vi "MyrioProject.vi"() -> ()   [LabVIEW 2018]
doc: "The myRIO Project template acquires acceleration data from the onboard accelerometer and displays the changes of acceleration values in a waveform chart."
uses:
  <vilib>/myRIO/Common/Instrument Driver Framework/Utilities/typedefs/Generic FPGA Reference.ctl
  <vilib>/myRIO/Common/Instrument Driver Framework/Utilities/typedefs/myRIO v1.0 Reference.ctl
  <vilib>/myRIO/Common/Instrument Driver Framework/Utilities/typedefs/Hardware Version Enum.ctl
  <vilib>/myRIO/Common/Instrument Driver Framework/Utilities/typedefs/myRIO Generic Hardware Reference.ctl
  <vilib>/userdefined/High Color/nirio_resource_hc.ctl
  <vilib>/myRIO/Common/Instrument Driver Framework/myRIO v1.0/Encoder/typedefs/Encoder Channels Enum.ctl
  <vilib>/myRIO/Instrument Drivers/Onboard IO/Encoder/typedefs/Encoder Reference.ctl
  <vilib>/myRIO/Instrument Drivers/Onboard IO/Encoder/Encoder.lvlib
  <vilib>/myRIO/Common/Instrument Driver Framework/myRIO v1.0/Encoder/typedefs/Encoder Signal Mode.ctl
  <vilib>/myRIO/Instrument Drivers/Onboard IO/Encoder/vis/myRIO Encoder Open.xnode
  <vilib>/myRIO/Common/Instrument Driver Framework/myRIO v1.0/Encoder/vis/myRIO v1.1 Open Encoder.vi
  <vilib>/myRIO/Common/Instrument Driver Framework/myRIO v1.0/Encoder/vis/myRIO v1.0 Configure Encoder.vi
  <vilib>/myRIO/Common/Instrument Driver Framework/myRIO v1.0/Encoder/typedefs/Encoder Configuration v1.0.ctl
  <vilib>/myRIO/Instrument Drivers/Onboard IO/PWM/typedefs/PWM Configuration.ctl
  <vilib>/myRIO/Instrument Drivers/Onboard IO/PWM/PWM.lvlib
  <vilib>/myRIO/Common/Instrument Driver Framework/myRIO v1.0/PWM/typedefs/PWM Channels Enum.ctl
  <vilib>/myRIO/Instrument Drivers/Onboard IO/PWM/typedefs/PWM Reference.ctl
  <vilib>/myRIO/Instrument Drivers/Onboard IO/PWM/vis/myRIO PWM Open.xnode
  <vilib>/myRIO/Common/Instrument Driver Framework/myRIO v1.0/PWM/vis/myRIO v1.1 Open PWM.vi
  <vilib>/myRIO/Express VI/Onboard Devices/Button/Button Express VI.xnode
  <vilib>/myRIO/Instrument Drivers/Onboard IO/DIO/typedefs/DIO Reference.ctl
  <vilib>/myRIO/Instrument Drivers/Onboard IO/DIO/DIO.lvlib
  <vilib>/myRIO/Common/Instrument Driver Framework/myRIO v1.0/DIO/typedefs/DIO Channels List.ctl
  <vilib>/myRIO/Common/Instrument Driver Framework/myRIO v1.0/DIO/typedefs/DIO Channels Enum.ctl
  <vilib>/myRIO/Instrument Drivers/Onboard IO/DIO/vis/myRIO DIO Open.xnode
  <vilib>/myRIO/Common/Instrument Driver Framework/myRIO v1.0/DIO/vis/myRIO v1.1 Open DIO.vi
  <vilib>/myRIO/Common/Instrument Driver Framework/Utilities/vis/Is FPGA Ref Available.vi
  <vilib>/myRIO/Express VI/Onboard IO/DO/DO Express VI.xnode
  <vilib>/myRIO/Instrument Drivers/Onboard IO/DIO/vis/Write.vi
  <vilib>/myRIO/Express VI/Onboard IO/AI/AI Express VI.xnode
  <vilib>/myRIO/Instrument Drivers/Onboard IO/AI/typedefs/AI Reference.ctl
  <vilib>/myRIO/Instrument Drivers/Onboard IO/AI/AI.lvlib
  <vilib>/myRIO/Common/Instrument Driver Framework/Utilities/typedefs/Analog Scaling Constants List.ctl
  <vilib>/myRIO/Common/Instrument Driver Framework/Utilities/typedefs/Analog Scaling Constants.ctl
  <vilib>/myRIO/Common/Instrument Driver Framework/myRIO v1.0/AI/typedefs/AI Channels List.ctl
  <vilib>/myRIO/Common/Instrument Driver Framework/myRIO v1.0/AI/typedefs/AI Channels Enum.ctl
  <vilib>/myRIO/Instrument Drivers/Onboard IO/AI/vis/myRIO AI Open.xnode
  <vilib>/myRIO/Common/Instrument Driver Framework/myRIO v1.0/AI/vis/myRIO v1.1 Open AI.vi
  <vilib>/myRIO/Express VI/Onboard IO/PWM/PWM Express VI.xnode
  <vilib>/myRIO/Instrument Drivers/Onboard IO/PWM/vis/Set Duty Cycle and Frequency.vi
  <vilib>/platform/TimedLoop/XDataNode/XDataNode.xnode
  <vilib>/Platform/TimedLoop/XDataNode/timing_clust.ctl
  <vilib>/Platform/TimedLoop/XDataNode/XDNodeRunTimeDep.lvlib
  <vilib>/Platform/TimedLoop/XDataNode/wakeup.ctl
  <vilib>/Platform/TimedLoop/XDataNode/nitl_modes.ctl
panel:
  out "Numeric Control":dbl
  out "data":dbl
  out "Double 2":dbl
  out "Double":dbl
  out "sensor2 (A/AI2 (Pin 7))":dbl
  out "sensor1":dbl
  out "stallRojo (A/AI0 (Pin 3))":dbl
  out "stallBlanco (A/AI1 (Pin 5))":dbl
  in  "MANUAL 2":bool
  in  "Stop Button":bool
  in  "Start":bool
  out "element":dbl
  out "element 2":dbl
  out "subarray 2":dbl[][](array[numeric])
  out "subarray":dbl[][](array[numeric])
  out "vectores":dbl[][][](array[numeric])
  in  "saturacion":dbl=0.3
  in  "Duty Cycle 2":dbl(slide)=0.5 scale=0.05..0.1
  in  "Duty Cycle":dbl(slide)=0.5 scale=0.05..0.1
  in  "Reset Counter 2":bool
  in  "Reset Counter":bool
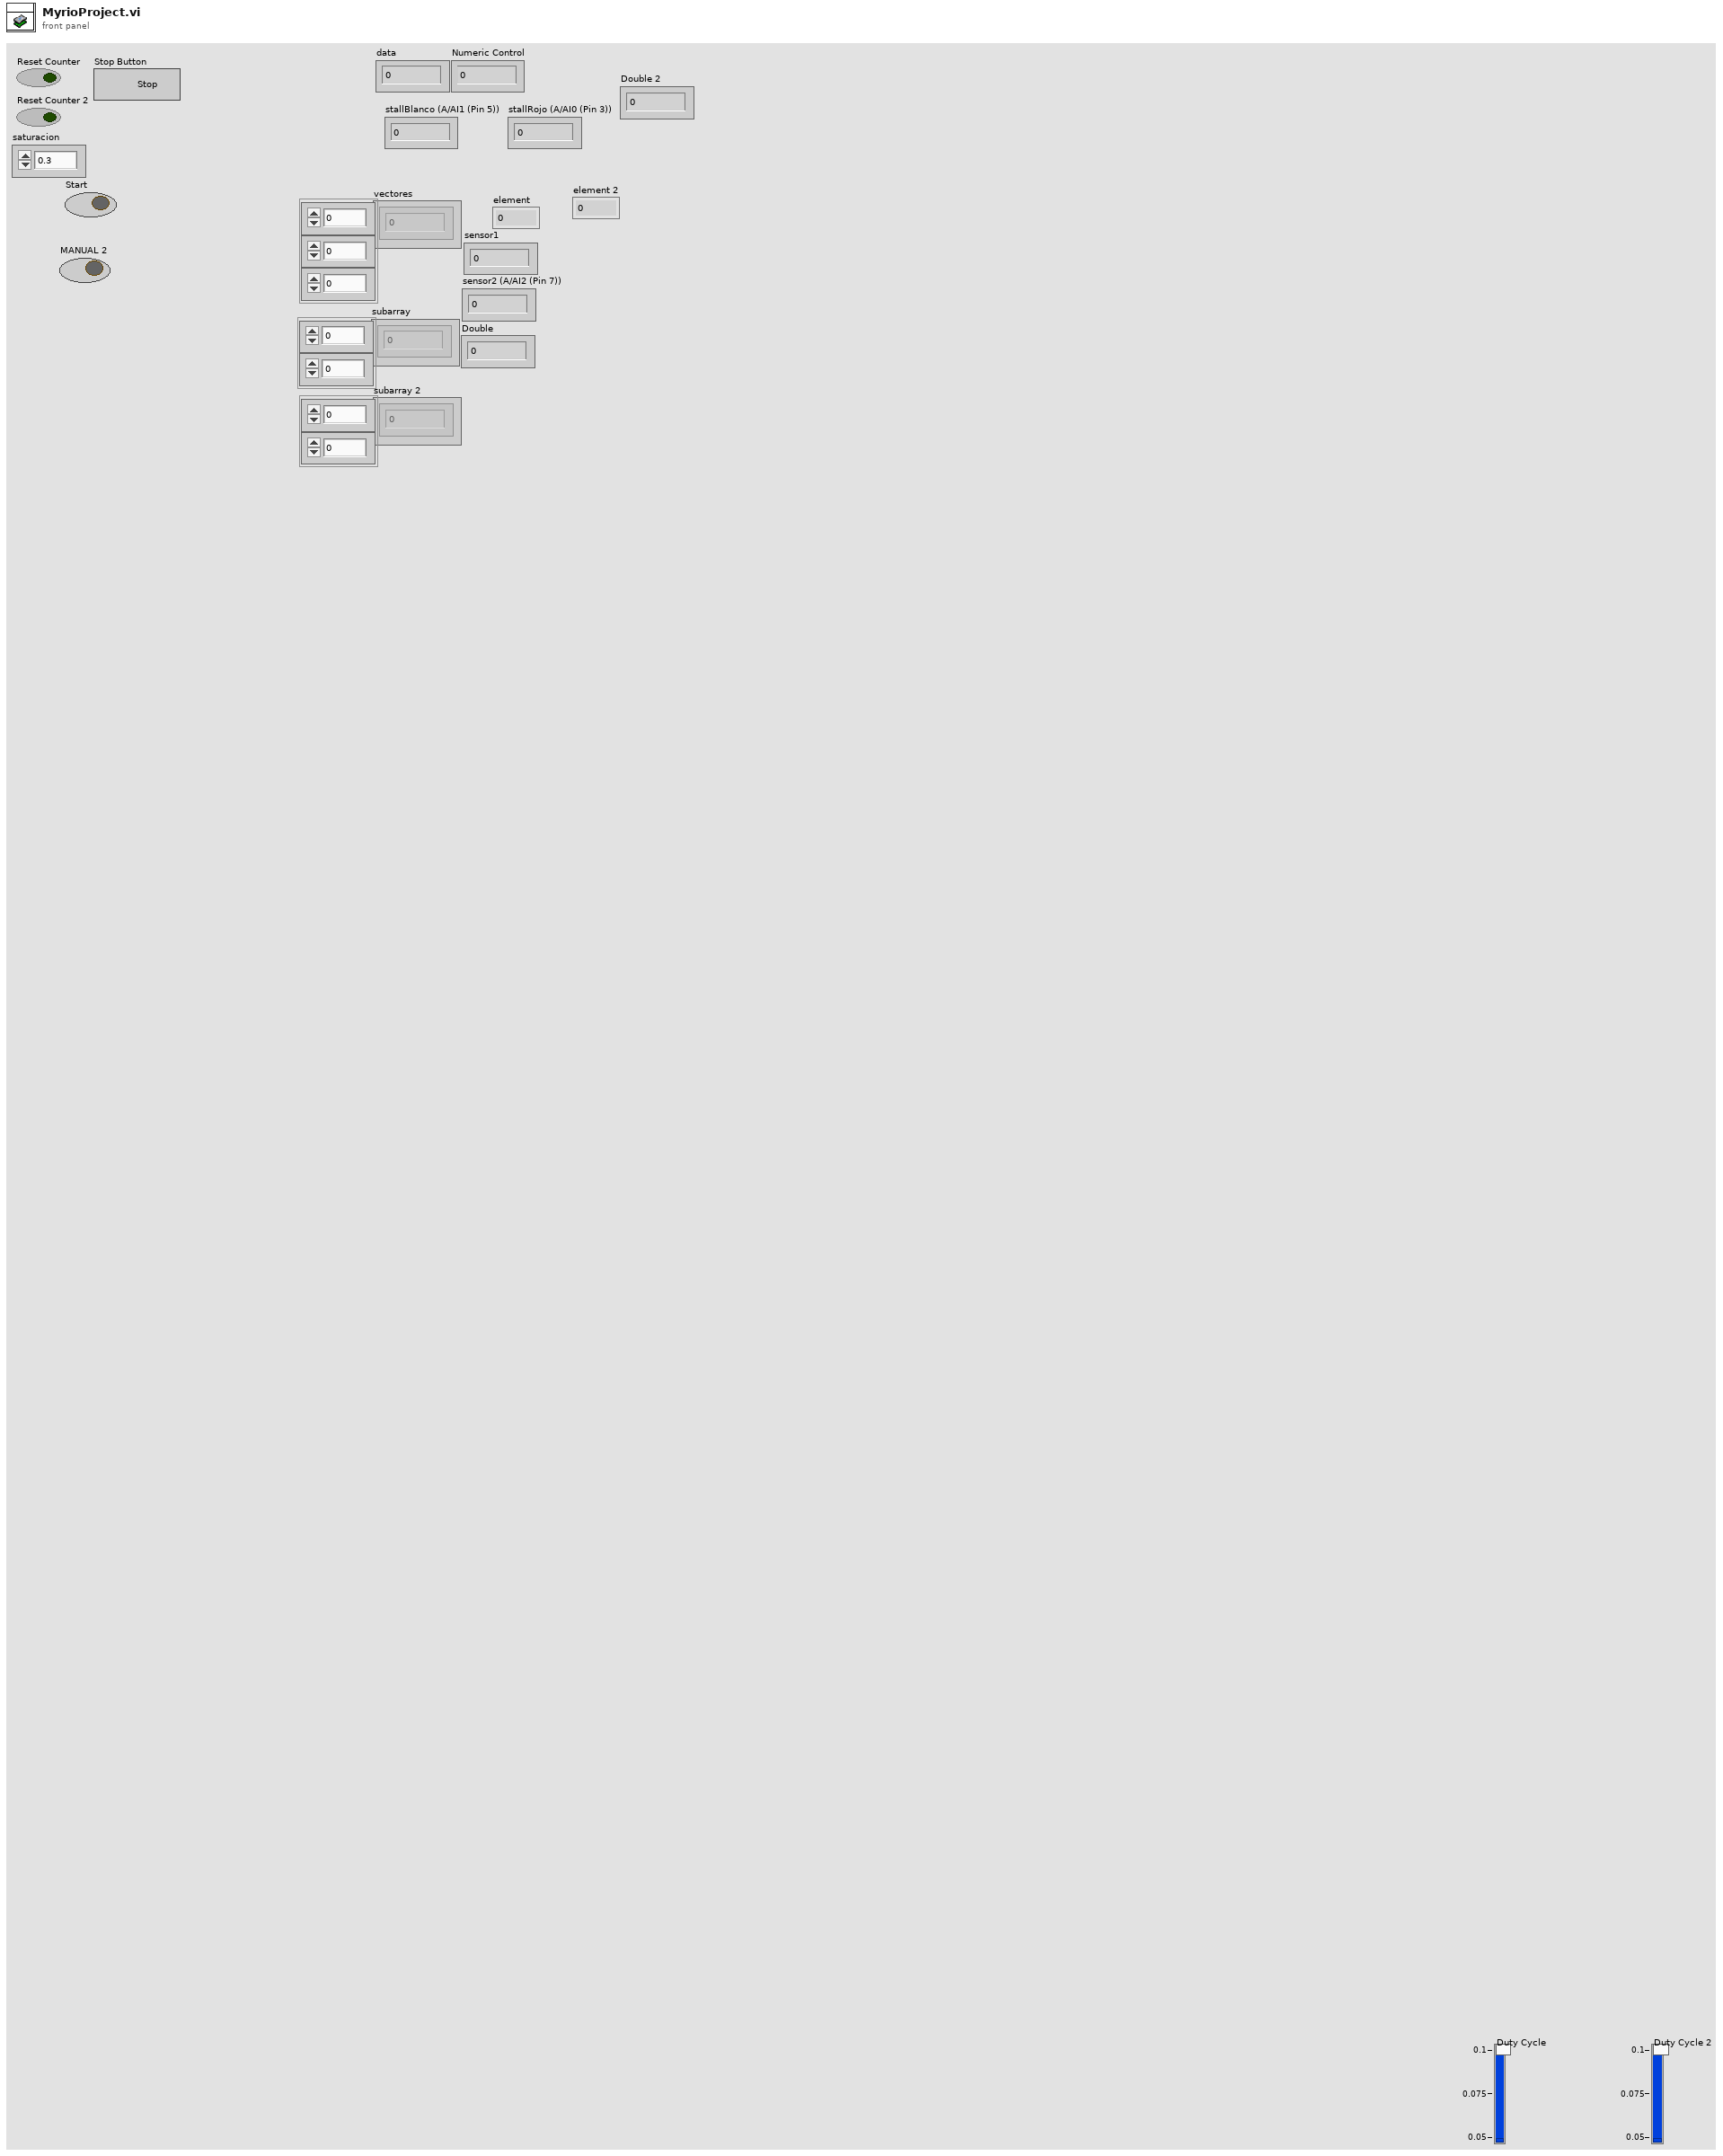
[diagram p1: front panel]
types:
  T1 = enum16{"normal", "grande-Sensor", "grande home", "peque-sensor", "peque- home", "peque-reset"}
  T2 = typedef "Encoder Signal Mode.ctl" = enum16{"Quadrature phase signal", "Step and direction signal"}
  T3 = typedef "PWM.lvlib/PWM Reference.ctl" = cluster{"myRIO Reference":T4, "PWM Channels Enum":T8, "PWM Configuration":T9}
  T4 = typedef "myRIO Generic Hardware Reference.ctl" = cluster{"myRIO Model":T5, "myRIO Hardware Reference":T6}
  T5 = typedef "Hardware Version Enum.ctl" = enum16{"Unknown", "myRIO-1900", "myRIO-1950", "roboRIO", "NI ELVIS RIO CM", "ELVIS III"}
  T6 = typedef "myRIO v1.0 Reference.ctl" = cluster{"Generic FPGA Reference":T7, "Allow multiple opens":bool}
  T7 = typedef "Generic FPGA Reference.ctl" = refnum<k20>
  T8 = typedef "PWM Channels Enum.ctl" = enum16{"Not Connected", "C/PWM0", "C/PWM1", "A/PWM0", "A/PWM1", "A/PWM2", "A/PWM3", "A/PWM4", "A/PWM5", "A/PWM6", "A/PWM7", "A/PWM8", "A/PWM9", "A/PWM10", "A/PWM11", "A/PWM12", "A/PWM13", "A/PWM14", "A/PWM15", "A/PWM16", "A/PWM17", "A/PWM18", "A/PWM19", "B/PWM0", "B/PWM1", "B/PWM2", "B/PWM3", "B/PWM4", "B/PWM5", "B/PWM6", "B/PWM7", "B/PWM8", "B/PWM9", "B/PWM10", "B/PWM11", "B/PWM12", "B/PWM13", "B/PWM14", "B/PWM15", "B/PWM16", "B/PWM17", "B/PWM18", "B/PWM19", "PWM/PWM0", "PWM/PWM1", "PWM/PWM2", "PWM/PWM3", "PWM/PWM4", "PWM/PWM5", "PWM/PWM6", "PWM/PWM7", "PWM/PWM8", "PWM/PWM9"}
  T9 = typedef "PWM.lvlib/PWM Configuration.ctl" = cluster{"Frequency":dbl, "Duty Cycle":dbl}
  T10 = typedef "Encoder.lvlib/Encoder Reference.ctl" = cluster{"myRIO Reference":T4, "Encoder Channels Enum":T11}
  T11 = typedef "Encoder Channels Enum.ctl" = enum16{"Not Connected", "C/ENC0", "C/ENC1", "A/ENC", "A/ENC0", "A/ENC1", "A/ENC2", "A/ENC3", "A/ENC4", "A/ENC5", "A/ENC6", "A/ENC7", "A/ENC8", "A/ENC9", "B/ENC", "B/ENC0", "B/ENC1", "B/ENC2", "B/ENC3", "B/ENC4", "B/ENC5", "B/ENC6", "B/ENC7", "B/ENC8", "B/ENC9", "DIO/ENC0", "DIO/ENC1", "DIO/ENC2", "DIO/ENC3", "DIO/ENC4"}
  T12 = cluster{"Double":dbl, "dbl Scaled Value":dbl, "Output":dbl, "seconds since 1Jan1904":timestamp, dbl, dbl, dbl}
  T13 = typedef "XDNodeRunTimeDep.lvlib/timing_clust.ctl" = cluster{"Expected End [f-1]":u64, "Actual End [f-1]":u64, "Finished Late? [f-1]":bool, "Expected End [i-1]":u64, "Actual End [i-1]":u64, "Finished Late? [i-1]":bool, "Expected Start [i]":u64, "Actual Start [i]":u64, "Expected Start [f]":u64, "Actual Start [f]":u64, "Source Name":string, "Structure Name":string, "Period":i64, "Deadline":i64, "Offset":i64, "Start":i64, "Priority":i32, "Timeout":i32, "Mode":T14, "Wakeup Reason":T15, "Error":errorcluster, "Source Type":string, "Secondary Source Type":string, "Global End Time":u64, "Global Start Time":u64, "Frame Duration":u64, "Iteration Duration":u64, "Assigned CPU":i32, "I/O Scan Engine Mode":u32}
  T14 = typedef "XDNodeRunTimeDep.lvlib/nitl_modes.ctl" = enum32{"No Change", "Process missed periods, maintain original phase", "Discard missed periods, maintain original phase", "Process missed periods, ignore original phase", "Discard missed periods, ignore original phase"}
  T15 = typedef "XDNodeRunTimeDep.lvlib/wakeup.ctl" = enum32{"Normal", "Aborted", "Asynchronous wakeup", "Timing source error", "Timed loop error", "Timeout"}
  T16 = typedef "nirio_resource_hc.ctl" = tag
  T17 = typedef "AI.lvlib/AI Reference.ctl" = cluster{"myRIO Reference":T4, "AI Channels List":T18, "AI Scaling Constants List":T20}
  T18 = typedef "AI Channels List.ctl" = T19[]
  T19 = typedef "AI Channels Enum.ctl" = enum16{"Not Connected", "AudioIn/Left", "AudioIn/Right", "C/AI0", "C/AI1", "A/AI0", "A/AI1", "A/AI2", "A/AI3", "A/AI4", "A/AI5", "A/AI6", "A/AI7", "B/AI0", "B/AI1", "B/AI2", "B/AI3", "B/AI4", "B/AI5", "B/AI6", "B/AI7", "AI/AI0", "AI/AI1", "AI/AI2", "AI/AI3", "A/AI0 (DIFF)", "A/AI1 (DIFF)", "A/AI2 (DIFF)", "A/AI3 (DIFF)", "B/AI0 (DIFF)", "B/AI1 (DIFF)", "B/AI2 (DIFF)", "B/AI3 (DIFF)"}
  T20 = typedef "Analog Scaling Constants List.ctl" = T21[]
  T21 = typedef "Analog Scaling Constants.ctl" = cluster{"LSB Weight (Volts)":dbl, "Offset (Volts)":dbl, "Signed?":bool}
  T22 = typedef "DIO.lvlib/DIO Reference.ctl" = cluster{"myRIO Reference":T4, "DIO Channels List":T23}
  T23 = typedef "DIO Channels List.ctl" = T24[]
  T24 = typedef "DIO Channels Enum.ctl" = enum16{"Not Connected", "C/DIO0", "C/DIO1", "C/DIO2", "C/DIO3", "C/DIO4", "C/DIO5", "C/DIO6", "C/DIO7", "A/DIO0", "A/DIO1", "A/DIO2", "A/DIO3", "A/DIO4", "A/DIO5", "A/DIO6", "A/DIO7", "A/DIO8", "A/DIO9", "A/DIO10", "A/DIO11", "A/DIO12", "A/DIO13", "A/DIO14", "A/DIO15", "A/DIO16", "A/DIO17", "A/DIO18", "A/DIO19", "B/DIO0", "B/DIO1", "B/DIO2", "B/DIO3", "B/DIO4", "B/DIO5", "B/DIO6", "B/DIO7", "B/DIO8", "B/DIO9", "B/DIO10", "B/DIO11", "B/DIO12", "B/DIO13", "B/DIO14", "B/DIO15", "B/DIO16", "B/DIO17", "B/DIO18", "B/DIO19", "LED0", "LED1", "LED2", "LED3", "Button0", "DIO/DIO0", "DIO/DIO1", "DIO/DIO2", "DIO/DIO3", "DIO/DIO4", "DIO/DIO5", "DIO/DIO6", "DIO/DIO7", "DIO/DIO8", "DIO/DIO9", "SPI/CS0", "SPI/CS1", "SPI/CS2", "SPI/CS3", "LED RADIO (Green)", "LED RADIO (Red)", "LED COMM (Green)", "LED COMM (Red)", "LED MODE (Green)", "LED MODE (Red)"}
  T25 = cluster{dbl, void, "Counter Value":i32, "seconds since 1Jan1904":timestamp, dbl, "saturacion":dbl, "Counter Value":i32}
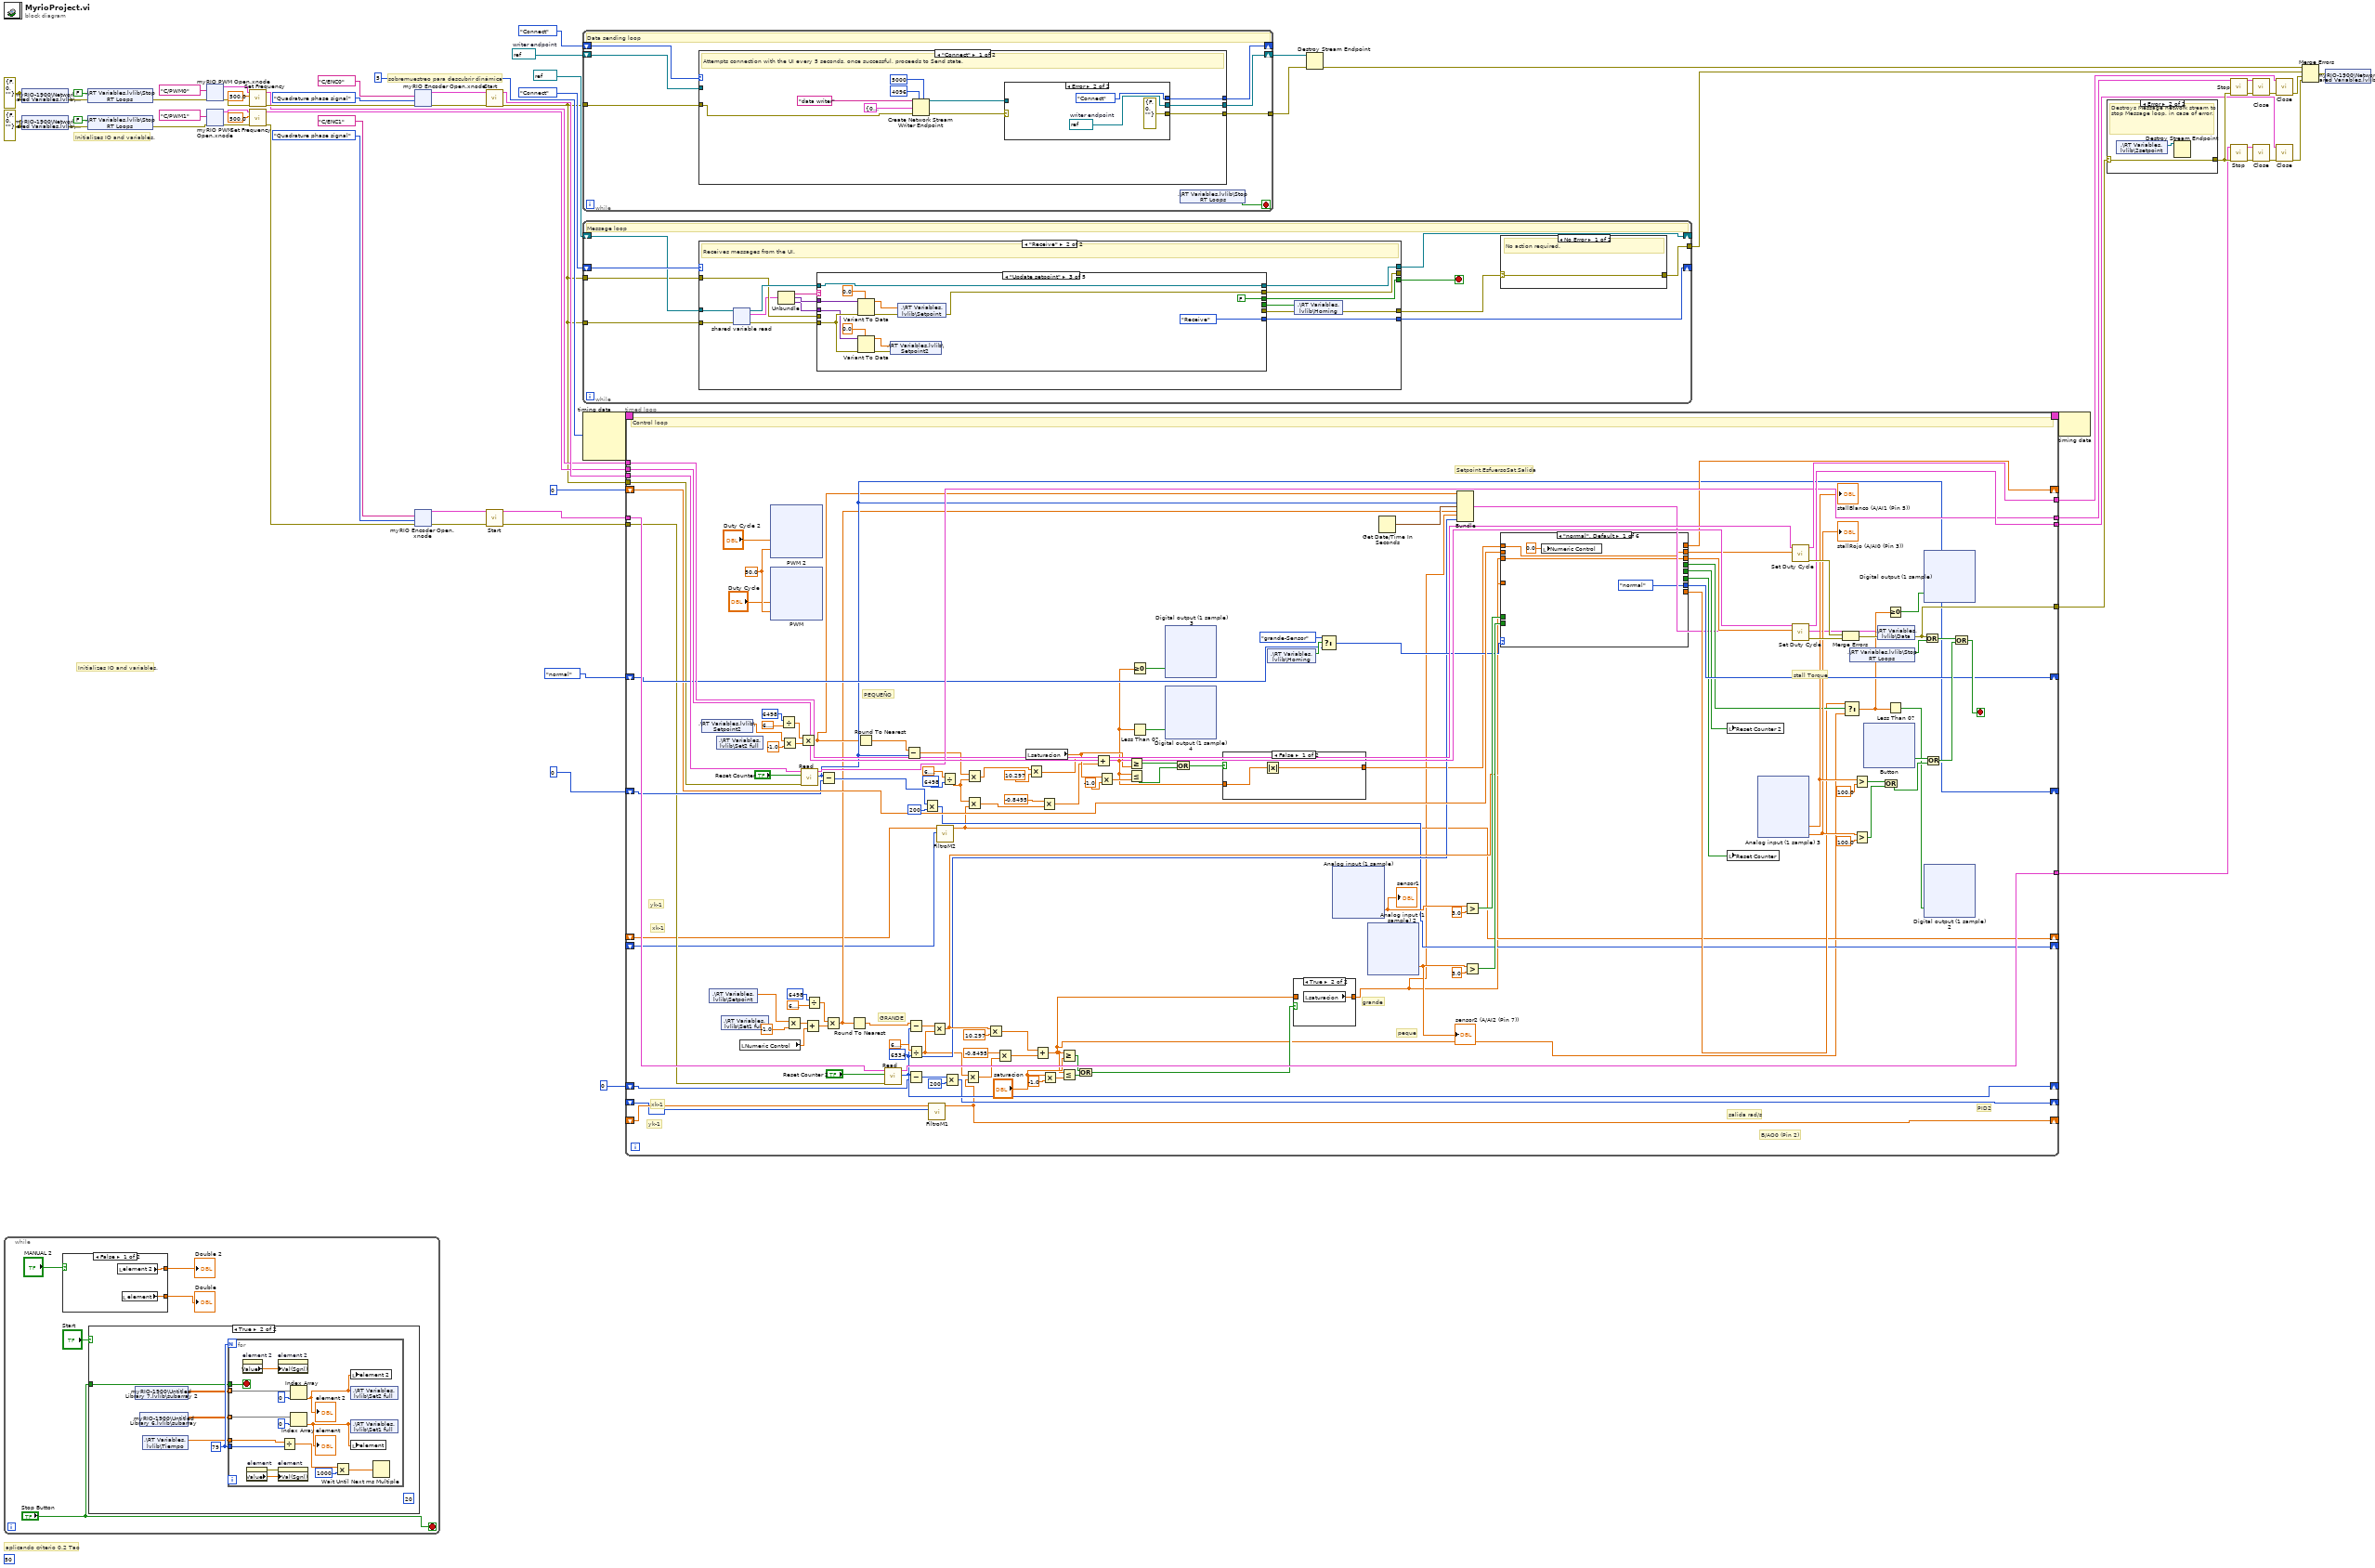
[diagram p0: block diagram]
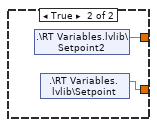
[diagram p2: hidden frame]
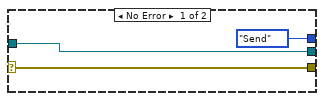
[diagram p5: hidden frame]
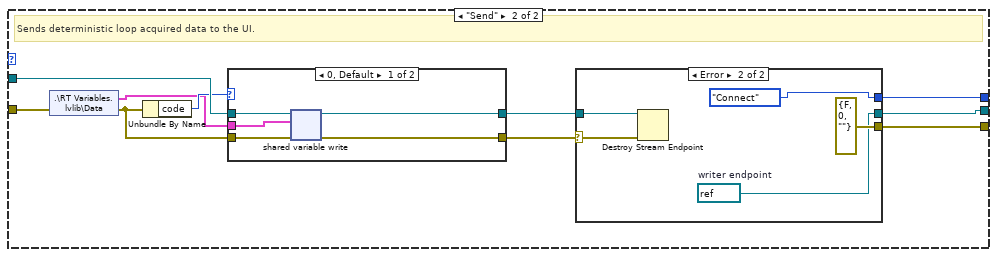
[diagram p6: hidden frame]
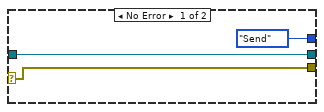
[diagram p7: hidden frame]
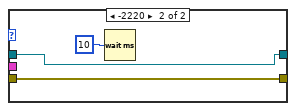
[diagram p8: hidden frame]
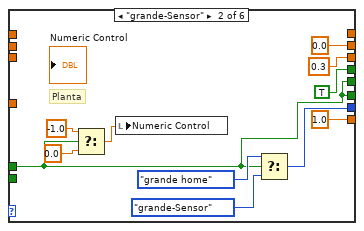
[diagram p9: hidden frame]
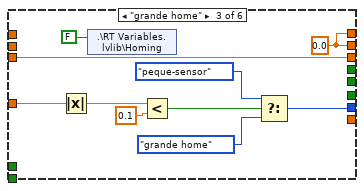
[diagram p10: hidden frame]
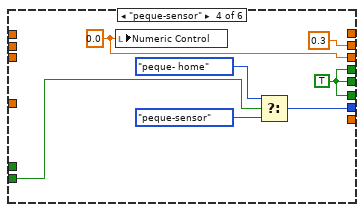
[diagram p11: hidden frame]
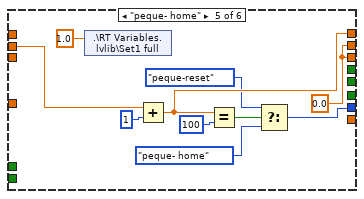
[diagram p12: hidden frame]
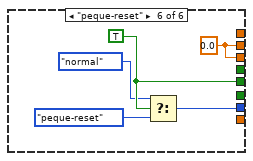
[diagram p13: hidden frame]
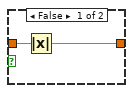
[diagram p14: hidden frame]
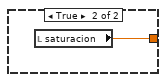
[diagram p15: hidden frame]
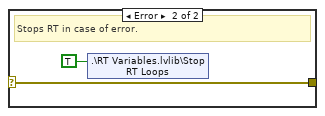
[diagram p16: hidden frame]
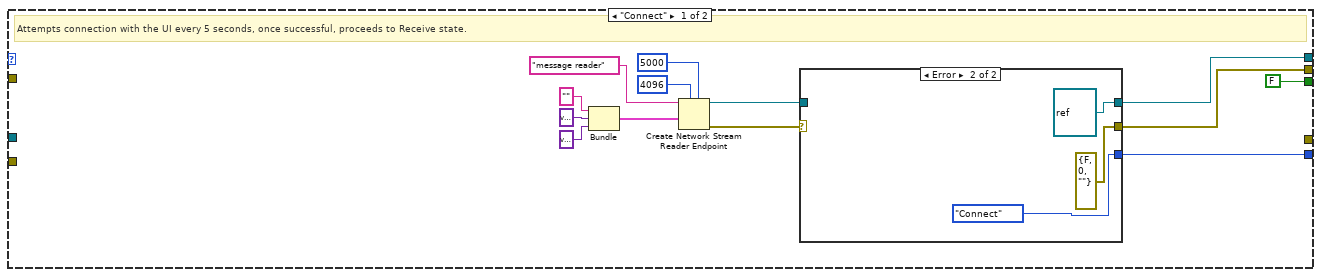
[diagram p17: hidden frame]
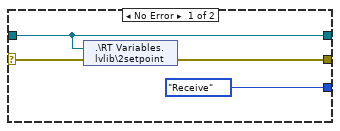
[diagram p18: hidden frame]
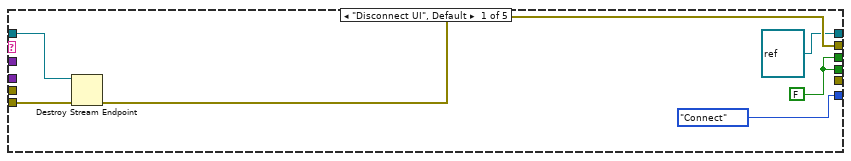
[diagram p19: hidden frame]
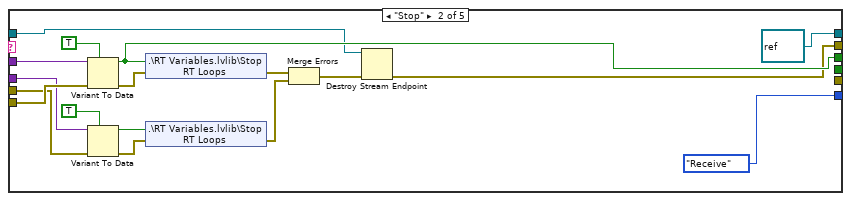
[diagram p20: hidden frame]
diagram:
  (unwired) 50
  w16 = refnum<k21> refnum  # writer endpoint
  w29 = errorcluster {"status"=FALSE, "code"=0, "source"=""} ("error IO")
  w51 = errorcluster {"status"=FALSE, "code"=0, "source"=""} ("error IO")
  # "aplicando criterio 0.2 Tao"
  # "sobremuestreo para descubrir dinámica"
  # "Initializes IO and variables."
  # "Initializes IO and variables."
  n1 = while {
    stop <- "Stop Button" stop-if-true
    n2 = case shown="False" "MANUAL 2" {
      tunnel: [w69 w71] -> w63
      tunnel: [w68 w70] -> w64
      frame False {
        n3 = local read "element 2"() -> (w69:dbl)
        n4 = local read "element"() -> (w68:dbl)
      }
      frame True {
        n5 = shared-variable ".\\RT Variables.lvlib\\Setpoint2"() -> (w71:dbl)  [unwired: 1 in, 1 out]
        n6 = shared-variable ".\\RT Variables.lvlib\\Setpoint"() -> (w70:dbl)  [unwired: 1 in, 1 out]
      }
    }
    "Double" <- w64
    "Double 2" <- w63
    n7 = case shown="True" "Start" {
      tunnel: "Stop Button" -> [_ w73]
      frame False {
      }
      frame True {
        (unwired) 20
        w76 = 79
        n8 = shared-variable "myRIO-1900\\Untitled Library 7.lvlib\\subarray 2"() -> (w74:dbl[][])  [unwired: 1 in, 1 out]
        n9 = shared-variable "myRIO-1900\\Untitled Library 6.lvlib\\subarray"() -> (w75:dbl[][])  [unwired: 1 in, 1 out]
        n10 = shared-variable ".\\RT Variables.lvlib\\Tiempo"() -> (w72:dbl)  [unwired: 1 in, 1 out]
        n11 = for {
          N: w76 -> [_]
          tunnel: w76 -> [w89]
          tunnel: w75 -> [w88] mode=indexing
          tunnel: w72 -> [w86]
          tunnel: w74 -> [w84] mode=indexing
          tunnel: w73 -> [w79]
          stop <- w79 stop-if-true
          n12 = property on="element 2" class="DigNum (strict)"() -> ("Value"=w81:dbl)  [unwired: 2 in, 2 out]
          n13 = property on="element" class="DigNum (strict)"() -> (error out=w82:errorcluster, "Value"=w83:dbl)  [unwired: 2 in, 1 out]
          n14 = property on="element 2" class="DigNum (strict)"("Val(Sgnl)"=w81) -> ()  [unwired: 2 in, 2 out]
          n15 = property on="element" class="DigNum (strict)"(error in=w82, "Val(Sgnl)"=w83) -> ()  [unwired: 1 in, 2 out]
          n16 = Divide(x=w86, y=w89) -> (x/y=w91:dbl)
          n17 = Index Array(array=w84, index=0) -> (element=w77:dbl)
          "element 2" <- w77
          n18 = Index Array(array=w88, index=0) -> (element=w78:dbl)
          "element" <- w78
          n19 = Multiply(x=w91, y=1000) -> (x*y=w80:dbl)
          n20 = local write "element 2"(w77) -> ()
          n21 = shared-variable ".\\RT Variables.lvlib\\Set2 full"(w77) -> ()  [unwired: 1 in, 1 out]
          n22 = shared-variable ".\\RT Variables.lvlib\\Set1 full"(w78) -> ()  [unwired: 1 in, 1 out]
          n23 = local write "element"(w78) -> ()
          n24 = Wait Until Next ms Multiple(millisecond multiple=w80) -> ()  [unwired: 1 out]
        }
      }
    }
  }
  n25 = shared-variable "myRIO-1900\\Network Shared Variables.lvlib\\error IO"(w51, error in=w51) -> (error out=w52:errorcluster)
  n26 = shared-variable "myRIO-1900\\Network Shared Variables.lvlib\\error IO"(w29, error in=w29) -> (error out=w30:errorcluster)
  n27 = shared-variable ".\\RT Variables.lvlib\\Stop RT Loops"(FALSE ("Stop RT Loops"), error in=w52) -> (error out=w39:errorcluster)
  n28 = shared-variable ".\\RT Variables.lvlib\\Stop RT Loops"(FALSE ("Stop RT Loops"), error in=w30) -> (error out=w22:errorcluster)
  n29 = xnode "myRIO PWM Open.xnode"("error in (no error)"=w39, "Channel Name"=tag "C/PWM0") -> ("error out"=w41:errorcluster, "PWM Ref Out"=w40:T3)  [unwired: 1 in]
  n30 = xnode "myRIO PWM Open.xnode"("error in (no error)"=w22, "Channel Name"=tag "C/PWM1") -> ("error out"=w24:errorcluster, "PWM Ref Out"=w23:T3)  [unwired: 1 in]
  n31 = call <vilib>:"Set Frequency.vi"("error in (no error)"=w41, "Frequency [Hz]"=500.0, "PWM Ref In"=w40) -> ("error out"=w38:errorcluster, "PWM Ref Out"=w35:T3)  [unwired: 6 in]
  n32 = call <vilib>:"Set Frequency.vi"("error in (no error)"=w24, "Frequency [Hz]"=500.0, "PWM Ref In"=w23) -> ("error out"=w21:errorcluster, "PWM Ref Out"=w17:T3)  [unwired: 6 in]
  n33 = xnode "myRIO Encoder Open.xnode"("error in (no error)"=w38, "Channel Name"=tag "C/ENC0", "Encoder Signal Mode"=Encoder_Signal_Mode."Quadrature phase signal") -> ("error out"=w48:errorcluster, "Encoder Ref Out"=w47:T10)  [unwired: 2 in]
  n34 = xnode "myRIO Encoder Open.xnode"("error in (no error)"=w21, "Channel Name"=tag "C/ENC1", "Encoder Signal Mode"=Encoder_Signal_Mode."Quadrature phase signal") -> ("error out"=w27:errorcluster, "Encoder Ref Out"=w26:T10)  [unwired: 2 in]
  n35 = call <vilib>:"Start.vi"("error in (no error)"=w48, "Encoder Ref In"=w47) -> ("error out"=w6:errorcluster, "Encoder Ref Out"=w45:T10)  [unwired: 8 in]
  n36 = call <vilib>:"Start.vi"("error in (no error)"=w27, "Encoder Ref In"=w26) -> ("error out"=w5:errorcluster, "Encoder Ref Out"=w18:T10)  [unwired: 8 in]
  n37 = while {
    shift-right: [w96] -> w57
    shift-left: w16 -> [w94]
    tunnel: [w95] -> w58
    tunnel: w6 -> [w93]
    shift-right: [w92] -> _
    shift-left: enum16{"Connect", "Send"}."Connect" ("Message states") -> [w97]
    stop <- w98 stop-if-true
    # "Data sending loop"
    n38 = case shown="\"Connect\"" w97 {
      tunnel: [w102 w117] -> w95
      tunnel: [w100 w115] -> w96
      tunnel: [w106 w118] -> w92
      tunnel: w94 -> [_ w124]
      tunnel: w93 -> [w103 w123]
      frame "Connect" {
        # "Attempts connection with the UI every 5 seconds, once successful, proceeds to Send state."
        n39 = Create Network Stream Writer Endpoint(5:5000 ("timeout in ms (-1)"), 7:4096 ("writer buffer size"), 8:w103, 9:T12 {"Double"=0.0, "dbl Scaled Value"=0.0, "Output"=0.0, "seconds since 1Jan1904"=timestamp(0 s since 1904-01-01), 0.0, 0.0, 0.0} ("Data"), 11:"data writer" ("writer name")) -> (0:w104:errorcluster, 3:w101:refnum<k21>)  [unwired: 2 in]
        n40 = case shown="Error" w104 {
          selector: w104 -> [w109 _]
          tunnel: [enum16{"Connect", "Send"}."Send" ("Message states") enum16{"Connect", "Send"}."Connect" ("Message states")] -> w106
          tunnel: [w109 errorcluster {"status"=FALSE, "code"=0, "source"=""} ("error IO")] -> w102
          tunnel: w101 -> [w111 _]
          tunnel: [w111 w112] -> w100
          frame No Error {
          }
          frame Error {
            w112 = refnum<k21> refnum  # writer endpoint
          }
        }
      }
      frame "Send" {
        # "Sends deterministic loop acquired data to the UI."
        n41 = shared-variable ".\\RT Variables.lvlib\\Data"(error in=w123) -> (w120:T12, error out=w122:errorcluster)
        n42 = Unbundle By Name(w122) -> ("code"=w121:i32)
        n43 = case shown="0, Default" w121 {
          tunnel: [w137 w139] -> w119
          tunnel: [w136 w138] -> w116
          tunnel: w124 -> [w135 w138]
          tunnel: w122 -> [w134 w139]
          tunnel: w120 -> [w133 _]
          frame 0, Default {
            n44 = shared-variable-write(w135, w134, w133) -> (w136:refnum<k21>, w137:errorcluster)  [unwired: 1 in, 1 out]
          }
          frame -2220 {
            n45 = Wait (ms)(milliseconds to wait=u32 10) -> ()  [unwired: 1 out]
          }
        }
        n46 = case shown="Error" w119 {
          selector: w119 -> [w127 w131]
          tunnel: [enum16{"Connect", "Send"}."Send" ("Message states") enum16{"Connect", "Send"}."Connect" ("Message states")] -> w118
          tunnel: [w127 errorcluster {"status"=FALSE, "code"=0, "source"=""} ("error IO")] -> w117
          tunnel: w116 -> [w125 w130]
          tunnel: [w125 w128] -> w115
          frame No Error {
          }
          frame Error {
            w128 = refnum<k21> refnum  # writer endpoint
            n47 = Destroy Stream Endpoint(8:w131, 11:w130) -> ()  [unwired: 1 out]
          }
        }
      }
    }
    n48 = shared-variable ".\\RT Variables.lvlib\\Stop RT Loops"() -> (w98:bool)  [unwired: 1 in, 1 out]
  }
  n49 = while {
    tunnel: [w144] -> w54
    shift-right: [w148] -> _
    shift-left: refnum<k21> refnum ("reader endpoint") -> [w146]
    shift-right: [w147] -> _
    shift-left: enum16{"Connect", "Receive"}."Connect" ("Message states") -> [w149]
    tunnel: w6 -> [w145]
    tunnel: w6 -> [w142]
    stop <- w143 stop-if-true
    # "Message loop"
    n50 = case shown="\"Receive\"" w149 {
      tunnel: [w156 w173] -> _
      tunnel: [w154 w185] -> w148
      tunnel: [w163 w182] -> w147
      tunnel: w146 -> [_ w181]
      tunnel: w145 -> [_ w184]
      tunnel: [FALSE ("Stop RT Loops") w183] -> w143
      tunnel: w142 -> [_ w178]
      tunnel: [_ w174] -> w141
      frame "Connect" {
        # "Attempts connection with the UI every 5 seconds, once successful, proceeds to Receive state."
        n51 = Bundle("", variant, variant) -> (w159:cluster{string, variant, variant})  [unwired: 1 in]
        n52 = Create Network Stream Reader Endpoint(5:5000 ("timeout in ms (-1)"), 7:4096 ("reader buffer size"), 9:w159, 11:"message reader" ("reader name")) -> (0:w158:errorcluster, 3:w153:refnum<k21>)  [unwired: 3 in]
        n53 = case shown="Error" w158 {
          selector: w158 -> [w168 _]
          tunnel: [enum16{"Connect", "Receive"}."Receive" ("Message states") enum16{"Connect", "Receive"}."Connect" ("Message states")] -> w163
          tunnel: [w167 errorcluster {"status"=FALSE, "code"=0, "source"=""} ("error IO")] -> w156
          tunnel: [w166 refnum<k21> refnum ("reader endpoint")] -> w154
          tunnel: w153 -> [w166 _]
          frame No Error {
            n54 = shared-variable ".\\RT Variables.lvlib\\2setpoint"(w166, error in=w168) -> (error out=w167:errorcluster)
          }
          frame Error {
          }
        }
      }
      frame "Receive" {
        # "Receives messages from the UI."
        n55 = shared-variable-read(w181, w184) -> (w180:refnum<k21>, w186:errorcluster, w177:cluster{string, variant, variant})  [unwired: 1 in, 1 out]
        n56 = Unbundle(w177) -> (w188:string, w187:variant, w179:variant)
        n57 = case shown="\"Update setpoint\"" w188 {
          tunnel: w187 -> [_ w209 w224 w230 w248]
          tunnel: w186 -> [w193 w211 w213 w229 w242]
          tunnel: [w192 w206 w220 w231 _] -> w173
          tunnel: [refnum<k21> refnum ("reader endpoint") refnum<k21> refnum ("reader endpoint") w219 w237 w246] -> w185
          tunnel: w180 -> [w191 w205 w219 w237 w246]
          tunnel: [w189 w208 FALSE ("Stop RT Loops") FALSE ("Stop RT Loops") FALSE ("Stop RT Loops")] -> w183
          tunnel: [enum16{"Connect", "Receive"}."Connect" ("Message states") enum16{"Connect", "Receive"}."Receive" ("Message states") enum16{"Connect", "Receive"}."Receive" ("Message states") enum16{"Connect", "Receive"}."Receive" ("Message states") enum16{"Connect", "Receive"}."Receive" ("Message states")] -> w182
          tunnel: w179 -> [_ w201 w212 w233 w241]
          tunnel: w178 -> [_ w200 _ _ _]
          tunnel: [w189 _ _ _ w239] -> w176
          tunnel: [_ _ _ _ w238] -> w175
          frame "Disconnect UI", Default {
            w189 = FALSE ("Stop RT Loops")
            n58 = Destroy Stream Endpoint(8:w193, 11:w191) -> (0:w192:errorcluster)
          }
          frame "Stop" {
            n59 = Variant To Data(error in=w211, type=TRUE ("Stop RT Loops"), Variant=w209) -> (data=w208:bool, error out=w210:errorcluster)
            n60 = Variant To Data(error in=w200, type=TRUE ("Stop RT Loops"), Variant=w201) -> (data=w198:bool, error out=w202:errorcluster)
            n61 = shared-variable ".\\RT Variables.lvlib\\Stop RT Loops"(w208, error in=w210) -> (error out=w196:errorcluster)
            n62 = shared-variable ".\\RT Variables.lvlib\\Stop RT Loops"(w198, error in=w202) -> (error out=w197:errorcluster)
            n63 = Merge Errors(w196, w197) -> (w195:errorcluster)
            n64 = Destroy Stream Endpoint(8:w195, 11:w205) -> (0:w206:errorcluster)
          }
          frame "Update setpoint" {
            n65 = Variant To Data(error in=w213, type=0.0, Variant=w224) -> (data=w222:dbl, error out=w221:errorcluster)
            n66 = Variant To Data(error in=w213, type=0.0, Variant=w212) -> (data=w215:dbl, error out=w214:errorcluster)
            n67 = shared-variable ".\\RT Variables.lvlib\\Setpoint2"(w215, error in=w214) -> ()  [unwired: 1 out]
            n68 = shared-variable ".\\RT Variables.lvlib\\Setpoint"(w222, error in=w221) -> (error out=w220:errorcluster)
          }
          frame "Vector Setpoints" {
            n69 = Variant To Data(error in=w229, type=0.0, Variant=w233) -> (data=w232:dbl)  [unwired: 1 out]
            n70 = Variant To Data(error in=w229, type=dbl[][][] [], Variant=w230) -> (data=w227:dbl[][][])  [unwired: 1 out]
            "vectores" <- w227
            n71 = Index Array(array=w227) -> (element #1=w226:dbl[][], element #2=w225:dbl[][])  [unwired: 6 in]
            "subarray" <- w226
            "subarray 2" <- w225
            n72 = shared-variable "myRIO-1900\\Untitled Library 6.lvlib\\subarray"(w226) -> ()  [unwired: 1 in, 1 out]
            n73 = shared-variable "myRIO-1900\\Untitled Library 7.lvlib\\subarray 2"(w225) -> ()  [unwired: 1 in, 1 out]
            n74 = shared-variable ".\\RT Variables.lvlib\\Tiempo"(w232) -> (error out=w231:errorcluster)  [unwired: 1 in]
          }
          frame "Homing" {
            n75 = Variant To Data(error in=w242, type=0.0, Variant=w241) -> (data=→"data":dbl)  [unwired: 1 out]
            n76 = Variant To Data(error in=w242, type=TRUE, Variant=w248) -> (data=w239:bool, error out=w238:errorcluster)
          }
        }
        n77 = shared-variable ".\\RT Variables.lvlib\\Homing"(w176, error in=w175) -> (error out=w174:errorcluster)
      }
    }
    n78 = case shown="No Error" w141 {
      selector: w141 -> [w150 w151]
      tunnel: [w150 w151] -> w144
      frame No Error {
        # "No action required."
      }
      frame Error {
        # "Stops RT in case of error."
        n79 = shared-variable ".\\RT Variables.lvlib\\Stop RT Loops"(TRUE ("Stop RT Loops")) -> ()  [unwired: 1 in, 1 out]
      }
    }
  }
  n80 = node-c288(i64 5 ("Period")) -> (w62:T13)  [unwired: 3 in]
  n81 = timed-loop {
    timing: w62 -> [_]
    timing-out: [_] -> w61
    tunnel: [w374] -> w50
    tunnel: w45 -> [w353]
    tunnel: [w352] -> w42
    tunnel: w35 -> [w341]
    tunnel: [w373] -> w34
    tunnel: w18 -> [w370]
    tunnel: w17 -> [w369]
    tunnel: [w365] -> w11
    tunnel: [w364] -> w10
    shift-right: [w339] -> _
    shift-left: T1."normal" ("Enum") -> [w338]
    shift-right: [w334] -> _
    shift-left: 0 -> [w333]
    shift-right: [w324] -> _
    shift-left: 0 -> [w325]
    tunnel: w5 -> [w319]
    tunnel: w6 -> [w318]
    shift-right: [w267] -> _
    shift-left: 0 ("Counter Value") -> [w266]
    shift-right: [w262] -> _
    shift-left: _ -> [w260]
    shift-right: [w259] -> _
    shift-left: _ -> [w261]
    shift-right: [w258] -> _
    shift-left: _ -> [w257]
    shift-right: [w255] -> _
    shift-left: _ -> [w256]
    stop <- w362 stop-if-true
    w321 = 50.0 ("Frequency [Hz]")
    # "yk-1"
    # "xk-1"
    # "yk-1"
    # "xk-1"
    # "PEQUEÑO"
    # "peque"
    # "grande"
    # "stall Torque"
    # "Setpoint,EsfuersoSat,Salida"
    # "PID2"
    # "GRANDE"
    # "salida rad/s"
    # "B/AO0 (Pin 2)"
    # "Control loop"
    n82 = shared-variable ".\\RT Variables.lvlib\\Setpoint2"() -> (w253:dbl)  [unwired: 1 in, 1 out]
    n83 = shared-variable ".\\RT Variables.lvlib\\Setpoint"() -> (w254:dbl)  [unwired: 1 in, 1 out]
    n84 = shared-variable ".\\RT Variables.lvlib\\Set2 full"() -> ()  [unwired: 1 in, 2 out]
    n85 = shared-variable ".\\RT Variables.lvlib\\Set1 full"() -> ()  [unwired: 1 in, 2 out]
    n86 = local read "Numeric Control"() -> (w287:dbl)
    n87 = xnode "PWM 2"("Duty Cycle"="Duty Cycle 2", "Frequency [Hz]"=w321) -> ()  [unwired: 1 in, 1 out]
    n88 = xnode "PWM"("Duty Cycle"="Duty Cycle", "Frequency [Hz]"=w321) -> ()  [unwired: 1 in, 1 out]
    n89 = Divide(x=6498, y=6.283185307179586) -> (x/y=w311:dbl)
    n90 = Multiply(x=w253, y=-1.0) -> (x*y=w283:dbl)
    n91 = Multiply(x=w254, y=-1.0) -> (x*y=w284:dbl)
    n92 = Multiply(x=w311, y=w283) -> (x*y=w279:dbl)
    n93 = call <vilib>:"Read.vi"("error in (no error)"=w318, "Reset Counter"="Reset Counter", "Encoder Ref In"=w353) -> ("Counter Value"=w324:i32, "Encoder Ref Out"=w352:T10)  [unwired: 4 in, 3 out]
    n94 = Add(x=w284, y=w287) -> (x+y=w285:dbl)
    n95 = Divide(x=6498, y=6.283185307179586) -> (x/y=w308:dbl)
    n96 = Subtract(x=w324, y=w325) -> (x-y=w297:i32)
    n97 = Multiply(x=w308, y=w285) -> (x*y=w276:dbl)
    n98 = Round To Nearest(number=w276) -> (nearest integer value=w356:dbl)
    n99 = Round To Nearest(number=w279) -> (nearest integer value=w351:dbl)
    n100 = call <vilib>:"Read.vi"("error in (no error)"=w319, "Reset Counter"="Reset Counter 2", "Encoder Ref In"=w370) -> ("Counter Value"=w267:i32, "Encoder Ref Out"=w365:T10)  [unwired: 4 in, 3 out]
    n101 = Subtract(x=w351, y=w324) -> (x-y=w326:dbl)
    n102 = Subtract(x=w356, y=w267) -> (x-y=w286:dbl)
    n103 = Subtract(x=w267, y=w266) -> (x-y=w269:i32)
    n104 = Divide(x=6.283185307179586, y=6534) -> (x/y=w265:dbl)
    n105 = Multiply(x=w297, y=200) -> (x*y=w258:i32)
    n106 = call "FiltroM1.vi"("Numeric 3"=w260, "Numeric in"=w261) -> ("Numeric out"=w259:dbl)  [unwired: 9 in]
    n107 = Multiply(x=w286, y=w265) -> (x*y=w273:dbl)
    n108 = call "FiltroM2.vi"("Numeric 3"=w257, "Numeric in"=w256) -> ("Numeric out"=w255:dbl)  [unwired: 9 in]
    n109 = Divide(x=6.283185307179586, y=6498) -> (x/y=w280:dbl)
    n110 = Multiply(x=w269, y=200) -> (x*y=w262:i32)
    n111 = Multiply(x=w265, y=w259) -> (x*y=w268:dbl)
    n112 = Multiply(x=w326, y=w280) -> (x*y=w294:dbl)
    n113 = Multiply(x=w280, y=w255) -> (x*y=w281:dbl)
    n114 = Multiply(x=w273, y=10.297) -> (x*y=w274:dbl)
    n115 = Multiply(x=-0.8495, y=w268) -> (x*y=w264:dbl)
    n116 = local read "saturacion"() -> (w303:dbl)
    n117 = Multiply(x=w294, y=10.297) -> (x*y=w327:dbl)
    n118 = Add(x=w274, y=w264) -> (x+y=w252:dbl)
    n119 = Multiply(x=-0.8495, y=w281) -> (x*y=w277:dbl)
    n120 = Multiply(x="saturacion", y=-1.0) -> (x*y=w302:dbl)
    n121 = Greater Or Equal?(x=w252, y="saturacion") -> (x >= y?=w359:bool)
    n122 = Less Or Equal?(x=w252, y=w302) -> (x <= y?=w358:bool)
    n123 = Or(x=w359, y=w358) -> (x .or. y?=w357:bool)
    n124 = Add(x=w327, y=w277) -> (x+y=w271:dbl)
    n125 = Multiply(x=w303, y=-1.0) -> (x*y=w305:dbl)
    n126 = Greater Or Equal?(x=w271, y=w303) -> (x >= y?=w361:bool)
    n127 = Less Or Equal?(x=w271, y=w305) -> (x <= y?=w360:bool)
    n128 = Greater Or Equal To 0?(x=w271) -> (x >= 0?=w307:bool)
    n129 = Less Than 0?(x=w271) -> (x < 0?=w306:bool)
    n130 = xnode "Digital output (1 sample) 3"("A/DIO2 (Pin 15)"=w307) -> ()  [unwired: 1 in, 1 out]
    n131 = xnode "Digital output (1 sample) 4"("A/DIO3 (Pin 17)"=w306) -> ()  [unwired: 1 in, 1 out]
    n132 = Or(x=w361, y=w360) -> (x .or. y?=w293:bool)
    n133 = case shown="False" w293 {
      tunnel: [w750 w751] -> w251
      tunnel: w271 -> [w749 _]
      frame False {
        n134 = Absolute Value(x=w749) -> (abs(x)=w750:dbl)
      }
      frame True {
        n135 = local read "saturacion"() -> (w751:dbl)
      }
    }
    n136 = shared-variable ".\\RT Variables.lvlib\\Homing"() -> (w342:bool)  [unwired: 1 in, 1 out]
    n137 = case shown="True" w357 {
      tunnel: [w746 w748] -> w250
      tunnel: w252 -> [w747 _]
      frame False {
        n138 = Absolute Value(x=w747) -> (abs(x)=w746:dbl)
      }
      frame True {
        n139 = local read "saturacion"() -> (w748:dbl)
      }
    }
    n140 = Select(t=T1."grande-Sensor" ("Enum"), s=w342, f=w338) -> (s? t:f=w291:T1)
    n141 = xnode "Analog input (1 sample)"() -> ("A/AI3 (Pin 9)"=w315:dbl)  [unwired: 1 in, 1 out]
    "sensor1" <- w315
    n142 = xnode "Analog input (1 sample) 2"() -> ("sensor2 (A/AI2 (Pin 7))"=w314:dbl)  [unwired: 1 in, 1 out]
    "sensor2 (A/AI2 (Pin 7))" <- w314
    n143 = Get Date/Time In Seconds() -> (seconds since 1Jan1904=w376:timestamp)
    n144 = Bundle(w279, "Counter Value"=w324, "seconds since 1Jan1904"=w376, w276, "saturacion"=w250, "Counter Value"=w267) -> (w278:T25, w249)  [unwired: 1 in]
    n145 = Greater?(x=w315, y=3.0) -> (0:w337:bool)
    n146 = Greater?(x=w314, y=3.0) -> (0:w335:bool)
    n147 = case shown="\"normal\", Default" w291 {
      tunnel: w251 -> [w450 _ _ _ _ _]
      tunnel: [w450 0.0 ("f") w468 0.3 ("f") w479 w493] -> w340
      tunnel: [T1."normal" ("Enum") w460 w471 w476 w485 w491] -> w339
      tunnel: w337 -> [_ w454 _ _ _ _]
      tunnel: w250 -> [w449 _ w467 _ _ _]
      tunnel: [w449 0.3 ("f") w467 w473 w479 w493] -> w336
      tunnel: w335 -> [_ _ _ w477 _ _]
      tunnel: [_ _ w468 _ w484 _] -> w334
      tunnel: w333 -> [_ _ _ _ w483 _]
      tunnel: [_ w454 _ w472 _ _] -> w331
      tunnel: [_ w454 _ w472 _ w490] -> w329
      tunnel: [_ 1.0 _ _ _ _] -> w288
      tunnel: [_ TRUE _ w472 _ _] -> w289
      tunnel: w273 -> [_ _ w466 _ _ _]
      frame "normal", Default {
        n148 = local write "Numeric Control"(0.0) -> ()
      }
      frame "grande-Sensor" {
        # "Planta"
        n149 = Select(t=-1.0, s=w454, f=0.0) -> (s? t:f=w451:dbl)
        n150 = local write "Numeric Control"(w451) -> ()
        n151 = Select(t=T1."grande home" ("Enum"), s=w454, f=T1."grande-Sensor" ("Enum")) -> (s? t:f=w460:T1)
      }
      frame "grande home" {
        w468 = 0.0
        n152 = Absolute Value(x=w466) -> (abs(x)=w465:dbl)
        n153 = shared-variable ".\\RT Variables.lvlib\\Homing"(FALSE ("Homing")) -> ()  [unwired: 1 in, 1 out]
        n154 = Less?(x=w465, y=0.1) -> (x < y?=w463:bool)
        n155 = Select(t=T1."peque-sensor" ("Enum"), s=w463, f=T1."grande home" ("Enum")) -> (s? t:f=w471:T1)
      }
      frame "peque-sensor" {
        w472 = TRUE
        w473 = 0.0 ("f")
        n156 = local write "Numeric Control"(w473) -> ()
        n157 = Select(t=T1."peque- home" ("Enum"), s=w477, f=T1."peque-sensor" ("Enum")) -> (s? t:f=w476:T1)
      }
      frame "peque- home" {
        w479 = 0.0 ("f")
        n158 = shared-variable ".\\RT Variables.lvlib\\Set1 full"(1.0) -> ()  [unwired: 1 in, 1 out]
        n159 = Add(x=w483, y=1) -> (x+y=w484:dbl)
        n160 = Equal?(x=w484, y=100) -> (x = y?=w488:bool)
        n161 = Select(t=T1."peque-reset" ("Enum"), s=w488, f=T1."peque- home" ("Enum")) -> (s? t:f=w485:T1)
      }
      frame "peque-reset" {
        w490 = TRUE
        w493 = 0.0 ("f")
        n162 = Select(t=T1."normal" ("Enum"), s=w490, f=T1."peque-reset" ("Enum")) -> (s? t:f=w491:T1)
      }
    }
    n163 = local write "Reset Counter 2"(w329) -> ()
    n164 = local write "Reset Counter"(w331) -> ()
    n165 = xnode "Analog input (1 sample) 3"() -> ("stallBlanco (A/AI1 (Pin 5))"=w317:dbl, "stallRojo (A/AI0 (Pin 3))"=w316:dbl)  [unwired: 1 in, 1 out]
    "stallBlanco (A/AI1 (Pin 5))" <- w317
    "stallRojo (A/AI0 (Pin 3))" <- w316
    n166 = call <vilib>:"Set Duty Cycle.vi"("Duty Cycle"=w340, "PWM Ref In"=w341) -> ("error out"=w367:errorcluster, "PWM Ref Out"=w373:T3)  [unwired: 7 in]
    n167 = call <vilib>:"Set Duty Cycle.vi"("Duty Cycle"=w336, "PWM Ref In"=w369) -> ("error out"=w368:errorcluster, "PWM Ref Out"=w364:T3)  [unwired: 7 in]
    n168 = Merge Errors(w367, w368) -> (w366:errorcluster)
    n169 = Select(t=w288, s=w289, f=w252) -> (s? t:f=w290:dbl)
    n170 = shared-variable ".\\RT Variables.lvlib\\Stop RT Loops"() -> (w375:bool)  [unwired: 1 in, 1 out]
    n171 = Greater?(x=w317, y=100.0) -> (0:w345:bool)
    n172 = Greater?(x=w316, y=100.0) -> (0:w344:bool)
    n173 = xnode "Button"() -> ("Value"=w323:bool)  [unwired: 1 in, 1 out]
    n174 = shared-variable ".\\RT Variables.lvlib\\Data"(w278, error in=w366) -> (error out=w374:errorcluster)
    n175 = Or(x=w345, y=w344) -> (x .or. y?=w346:bool)
    n176 = Greater Or Equal To 0?(x=w290) -> (x >= 0?=w299:bool)
    n177 = Less Than 0?(x=w290) -> (x < 0?=w298:bool)
    n178 = Or(x=w374, y=w375) -> (x .or. y?=w363:bool)
    n179 = xnode "Digital output (1 sample)"("A/DIO0 (Pin 11)"=w299) -> ()  [unwired: 1 in, 1 out]
    n180 = xnode "Digital output (1 sample) 2"("A/DIO1 (Pin 13)"=w298) -> ()  [unwired: 1 in, 1 out]
    n181 = Or(x=w323, y=w346) -> (x .or. y?=w343:bool)
    n182 = Or(x=w363, y=w343) -> (x .or. y?=w362:bool)
  }
  n183 = Destroy Stream Endpoint(8:w58, 11:w57) -> (0:w55:errorcluster)
  n184 = node-c288(w61) -> ()  [unwired: 1 out]
  n185 = case shown="Error" w50 {
    selector: w50 -> [w789 w790]
    tunnel: [w789 w790] -> w12
    frame No Error {
      # "No action required."
    }
    frame Error {
      # "Destroys Message network stream to stop Message loop, in case of error."
      n186 = shared-variable ".\\RT Variables.lvlib\\2setpoint"() -> (w791:refnum<k21>)  [unwired: 1 in, 1 out]
      n187 = Destroy Stream Endpoint(11:w791) -> ()  [unwired: 1 in, 1 out]
    }
  }
  n188 = call <vilib>:"Stop.vi"("error in (no error)"=w12, "Encoder Ref In"=w42) -> ("error out"=w43:errorcluster, "Encoder Ref Out"=w44:T10)  [unwired: 8 in]
  n189 = call <vilib>:"Stop.vi"("error in (no error)"=w12, "Encoder Ref In"=w11) -> ("error out"=w14:errorcluster, "Encoder Ref Out"=w15:T10)  [unwired: 8 in]
  n190 = call <vilib>:"Close.vi"("error in (no error)"=w43, "Encoder Ref In"=w44) -> ("error out"=w37:errorcluster)  [unwired: 9 in]
  n191 = call <vilib>:"Close.vi"("error in (no error)"=w14, "Encoder Ref In"=w15) -> ("error out"=w13:errorcluster)  [unwired: 9 in]
  n192 = call <vilib>:"Close.vi"("error in (no error)"=w37, "PWM Ref In"=w34) -> ("error out"=w36:errorcluster)  [unwired: 9 in]
  n193 = call <vilib>:"Close.vi"("error in (no error)"=w13, "PWM Ref In"=w10) -> ("error out"=w9:errorcluster)  [unwired: 9 in]
  n194 = Merge Errors(w55, w54, w36, w9) -> (w53:errorcluster)
  n195 = shared-variable "myRIO-1900\\Network Shared Variables.lvlib\\error IO"(w53) -> ()  [unwired: 1 in, 1 out]
